vi "Model - Get RT Status.vi"(8 "error in (no error)":errorcluster, 11 "View Model":T3) -> (0 "error out":errorcluster, 2 "RT Status":T1 {"Status NPL"."Duration, us" format="%0.2f"; "Status TCL2"."Duration, us" format="%0.2f"; "Status TCL1"."Duration, us" format="%0.2f"}, 3 "View Model":T3)   [LabVIEW 2017]
doc: "Get actual value of RT Status from DVR"
uses:
  Controls/View Model.ctl
  Controls/Shared Model.ctl
  Error Handler/Controls/Error Model.ctl
  Error Handler/Controls/Error Event.ctl
  Error Handler/Controls/Error Type.ctl
  Controller/Controls/Controller Model.ctl
  Controller/Controls/Controller Event.ctl
  Controller/Controls/Controller Command.ctl
  Controller/Controls/Controller Overhead.ctl
  Real-Time/RT Status.ctl
  Real-Time/RT Loop Status.ctl
  Controller/Controls/Controller Update Data.ctl
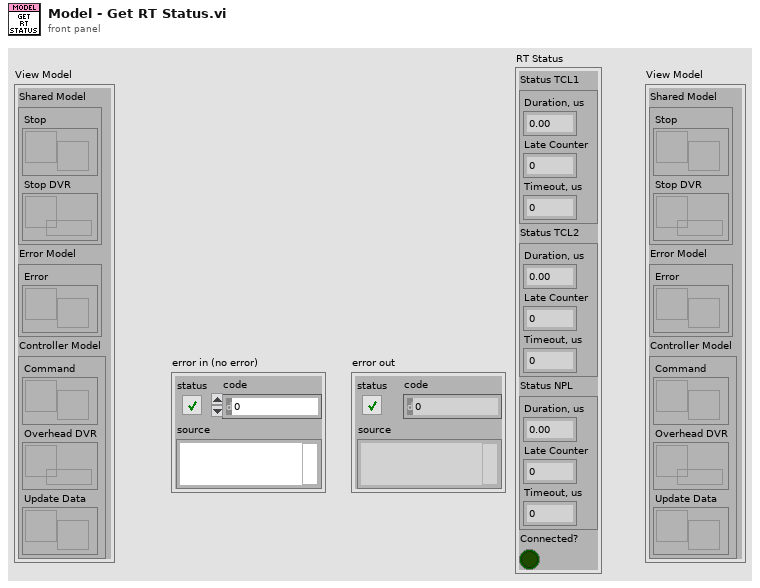
[diagram p1: front panel]
types:
  T1 = typedef "RT Status.ctl" = cluster{"Status TCL1":T2, "Status TCL2":T2, "Status NPL":T2, "Connected?":bool}
  T2 = typedef "RT Loop Status.ctl" = cluster{"Duration, us":dbl, "Late Counter":i32, "Timeout, us":u32}
  T3 = typedef "View Model.ctl" = cluster{"Shared Model":T4, "Error Model":T5, "Controller Model":T6}
  T4 = typedef "Shared Model.ctl" = cluster{"Stop":refnum<user-event>, "Stop DVR":refnum<data-value>}
  T5 = typedef "Error Model.ctl" = cluster{"Error":refnum<user-event>}
  T6 = typedef "Controller Model.ctl" = cluster{"Command":refnum<user-event>, "Overhead DVR":refnum<data-value>, "Update Data":refnum<user-event>}
  T7 = typedef "Controller Overhead.ctl" = cluster{"Start":bool, "Numeric":dbl, "Blink CNTRLR1":bool, "Blink CNTRLR2":bool, "RT Status":T1}
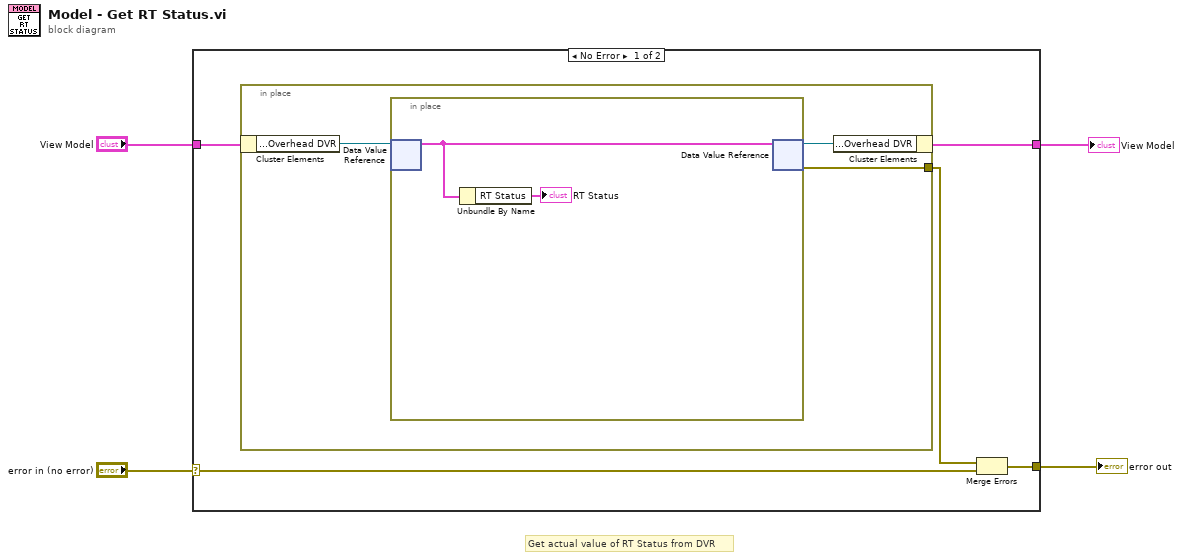
[diagram p0: block diagram]
diagram:
  # "Get actual value of RT Status from DVR"
  n1 = case shown="No Error" "error in (no error)" {
    selector: "error in (no error)" -> [w6 w15]
    tunnel: "View Model" -> [w9 w16]
    tunnel: [w8 w16] -> w2
    tunnel: [w5 w15] -> w1
    frame No Error {
      n2 = in-place {
        in-place-border: [w10] -> w7
        n3 = in-place-cluster #1(w9) -> ("Controller Model.Overhead DVR"=w12:refnum<data-value>)
        n4 = in-place {
          n5 = in-place-dvr #2(w12) -> (w14:T7)  [unwired: 1 out]
          n6 = Unbundle By Name(w14) -> ("RT Status"=→"RT Status":T1)
          n7 = in-place-dvr #2(w14) -> (w11:refnum<data-value>, w10:errorcluster)
        }
        n8 = in-place-cluster #1("Controller Model.Overhead DVR"=w11) -> (w8:T3)
      }
      n9 = Merge Errors(w7, w6) -> (w5:errorcluster)
    }
    frame Error {
    }
  }
  "View Model" <- w2
  "error out" <- w1
